vi "Temperature Controller (No Objects).vi"(8 "error in (no error)":errorcluster) -> (0 "error out":errorcluster, 3 "Temperature Controller out":refnum<class "Temperature Controller.lvclass">)   [LabVIEW 2009]
uses:
  Temperature Controller.lvclass
  Utility Classes/Readable/Channel Units.ctl
  Utility Classes/Readable/Readable.lvclass
  Global/GPIB Numbers.vi
  HV Slide Indicator.ctl
  AutoCtl.ctl
  Oxford/BUSGEN.LLB/OxfordAddress.ctl
  Oxford/ITCSUBS.LLB/ITCVersion.ctl
  Oxford/ITCSUBS.LLB/ITCIO.ctl
panel:
  in  "Cluster In":T6={"Heater"=0.0, "Needle Valve              (est. %)"=0.0, "PID Temp Setpoint"=0.0, "Auto"={"Auto Heater"=FALSE, "Auto Needle"=FALSE, "Auto PID"=FALSE}, "Needle Valve Timestamp"=0, "Needle Valve open/close rate (ms)"=66000, "Needle Valve Setpoint"=0.0, "ITC IO Info"={"Address"={"Com Port"=1, "ISOBUS Address"=1, "GPIB Address"=24, "Communication"=enum."ISOBUS"}, "Version"=enum."ITC503", "Ch 1 dec places"=1, "Ch 2 dec places"=1, "Ch 3 dec places"=1, "Ch1 Name"="Temperature", "Ch2 Name"="", "Ch3 Name"=""}} {"Heater" max=100.0 scale=0.0..100.0 scale format="%.1f"; "Needle Valve              (est. %)" max=100.0 scale=0.0..100.0 scale format="%.1f"; "Needle Valve Setpoint" max=100.0 scale=0.0..100.0 scale format="%.1f"}
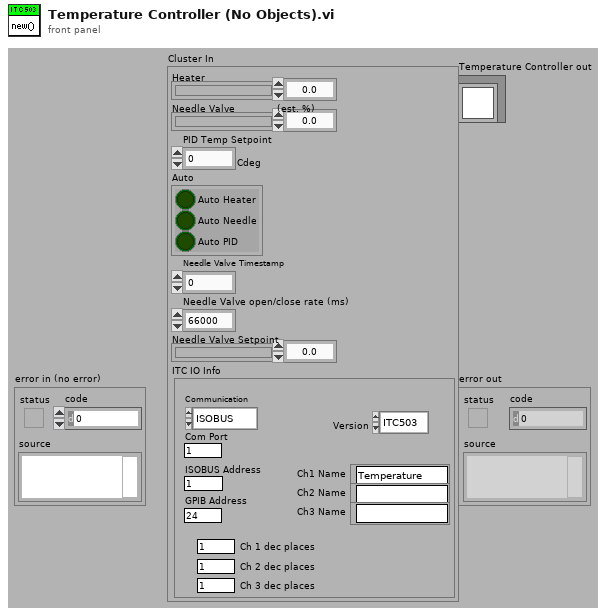
[diagram p1: front panel]
types:
  T1 = typedef "Temperature Controller.lvclass/HV Slide Indicator.ctl" = dbl
  T2 = typedef "Temperature Controller.lvclass/AutoCtl.ctl" = cluster{"Auto Heater":bool, "Auto Needle":bool, "Auto PID":bool}
  T3 = typedef "ITCIO.ctl" = cluster{"Address":T4, "Version":T5, "Ch 1 dec places":i16, "Ch 2 dec places":i16, "Ch 3 dec places":i16, "Ch1 Name":string, "Ch2 Name":string, "Ch3 Name":string}
  T4 = typedef "OxfordAddress.ctl" = cluster{"Com Port":i32, "ISOBUS Address":i32, "GPIB Address":i16, "Communication":enum16{"RS232", "ISOBUS", "GPIB", "Gateway"}}
  T5 = typedef "ITCVersion.ctl" = enum16{"ITC502", "ITC503", "ITC601"}
  T6 = cluster{"Heater":T1, "Needle Valve              (est. %)":T1, "PID Temp Setpoint":dbl[unit], "Auto":T2, "Needle Valve Timestamp":u32, "Needle Valve open/close rate (ms)":u32, "Needle Valve Setpoint":T1, "ITC IO Info":T3}
  T7 = typedef "Readable.lvclass/Channel Units.ctl" = string[]
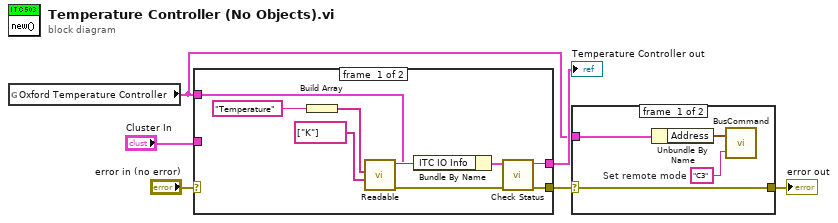
[diagram p0: block diagram]
diagram:
  n1 = global read "GPIB Numbers.vi" "Oxford Temperature Controller"() -> (w4:T3)
  n2 = case shown="No Error" "error in (no error)" {
    selector: "error in (no error)" -> [w14 w21]
    tunnel: [w16 w21] -> w3
    tunnel: [w17 w20] -> w5
    tunnel: "Cluster In" -> [w19 w20]
    tunnel: w4 -> [w7 _]
    frame #0 {
      n3 = Build Array("Temperature") -> (w8:string[])
      n4 = call "Readable.vi"("Channel Units"=T7 ["K"], "Channel Names"=w8) -> ("error out"=w11:errorcluster, "Readable out"=w13:refnum<class "Temperature Controller.lvclass">, "error in (no error)"=w12:errorcluster, "Readable in"=w15:refnum<class "Temperature Controller.lvclass">)  [unwired: 6 in]
      n5 = Bundle By Name(cluster=w13, "ITC IO Info"=w7) -> (w18:cluster{})
      n6 = call-dynamic "Check Status.vi"("error in (no error)"=w11, "Temperature Controller in"=w18) -> ("error out"=w16:errorcluster, "Temperature Controller out"=w17:refnum<class "Temperature Controller.lvclass">)  [unwired: 6 in, 2 out]
    }
    frame #1 {
    }
  }
  "Temperature Controller out" <- w5
  n7 = case shown="No Error" w3 {
    selector: w3 -> [w25 w26]
    tunnel: [w25 w26] -> w2
    tunnel: w4 -> [w22 _]
    frame #0 {
      w24 = "C3"  # Set remote mode
      n8 = Unbundle By Name(w22) -> ("Address"=w23:T4)
      n9 = call "BusCommand.vi"("Command"=w24, "Instrument address (in)"=w23) -> ()  [unwired: 2 out]
    }
    frame #1 {
    }
  }
  "error out" <- w2
